vi "Set Socket2.vi"(8 "error in (no error)":errorcluster, 11 "Channel Rep in":refnum<class "Channel Rep.lvclass">) -> (0 "error out":errorcluster, 3 "Channel Rep out":refnum<class "Channel Rep.lvclass">)   [LabVIEW 2018]
uses:
  Channel Rep/Channel Rep.lvclass
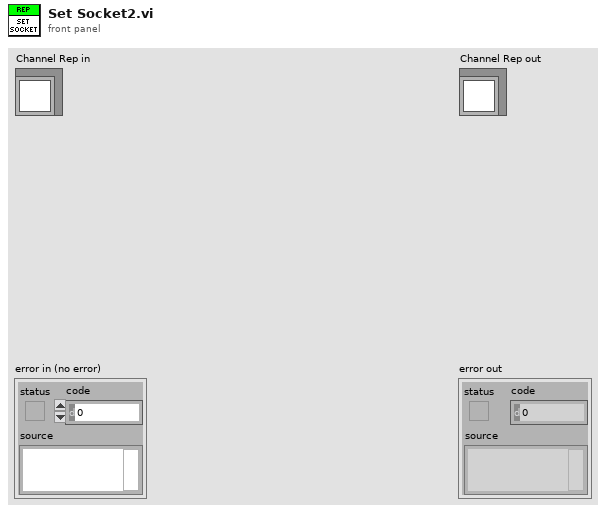
[diagram p1: front panel]
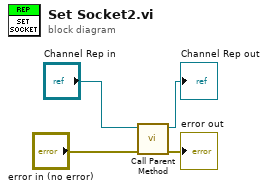
[diagram p0: block diagram]
diagram:
  n1 = call-parent "Call Parent Method"("error in (no error)"="error in (no error)", "Channel Pub in"="Channel Rep in") -> ("error out"=→"error out":errorcluster, "Channel Pub out"=→"Channel Rep out":refnum<class "Channel Rep.lvclass">)  [unwired: 8 in]
